vi "Leakge_Parse_Write.vi"(0 "LKG Path":path, 1 "Y2 axis on/off":bool, 2 "Y2 axis settings":T2, 3 "Vd Data":dbl[](array[numeric]), 5 "Var1 sweep settings":T3, 7 "Header in":string, 9 "Var2 step settings":T1, 11 "Vname 2":string, 12 "Execute?":bool, 13 "Vname":string, 14 "Y2 Output Cluster":cluster{"trace":dbl[], "trace":dbl[]}) -> ()   [LabVIEW 2012]
uses:
  <vilib>/Utility/file.llb/Write To Spreadsheet File (DBL).vi
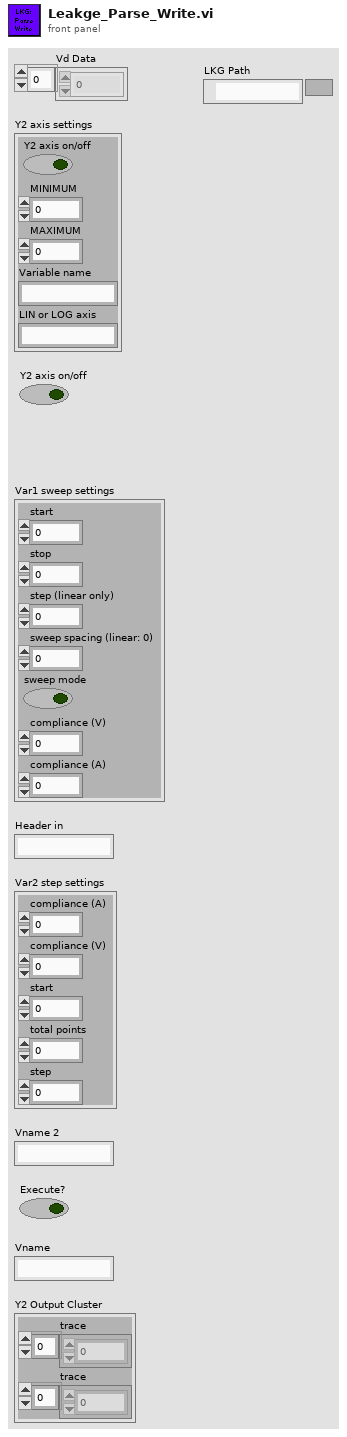
[diagram p1: front panel]
types:
  T1 = cluster{"compliance (A)":dbl, "compliance (V)":dbl, "start":dbl, "total points":u16, "step":dbl}
  T2 = cluster{"Y2 axis on/off":bool, "MINIMUM":ext, "MAXIMUM":ext, "Variable name":string, "LIN or LOG axis":string}
  T3 = cluster{"start":dbl, "stop":dbl, "step (linear only)":dbl, "sweep spacing (linear: 0)":u16, "sweep mode":bool, "compliance (V)":dbl, "compliance (A)":dbl}
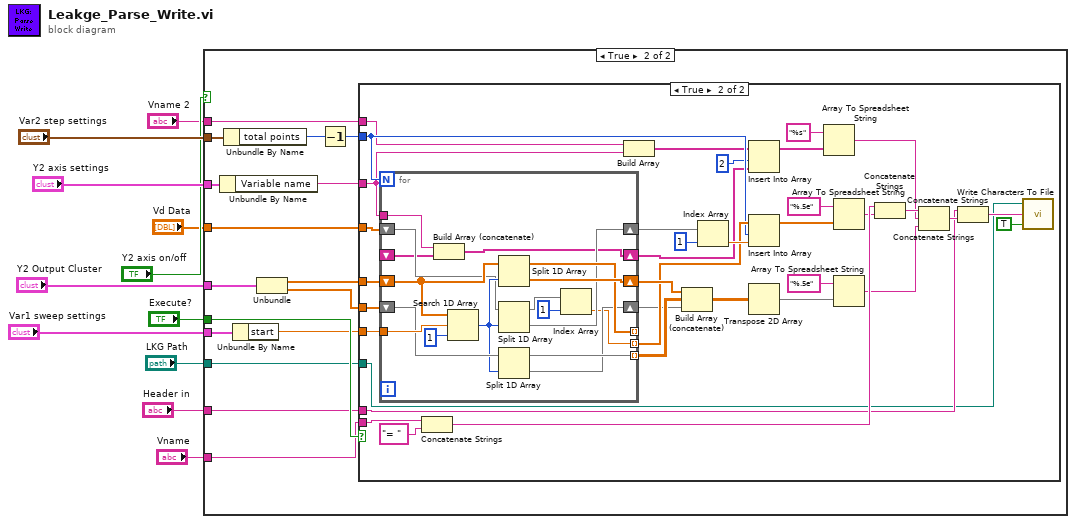
[diagram p0: block diagram]
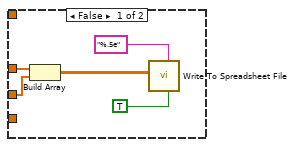
[diagram p3: hidden frame]
diagram:
  n1 = case shown="True" "Y2 axis on/off" {
    tunnel: "Execute?" -> [_ w27]
    tunnel: "Vd Data" -> [_ w26]
    tunnel: "Vname" -> [_ w25]
    tunnel: "Vname 2" -> [_ w24]
    tunnel: "Header in" -> [_ w23]
    tunnel: "LKG Path" -> [_ w22]
    tunnel: "Var2 step settings" -> [_ w21]
    tunnel: "Y2 axis settings" -> [_ w18]
    tunnel: "Var1 sweep settings" -> [_ w16]
    tunnel: "Y2 Output Cluster" -> [_ w14]
    frame False {
    }
    frame True {
      n2 = Unbundle By Name(w18) -> ("Variable name"=w17:string)
      n3 = Unbundle By Name(w21) -> ("total points"=w20:u16)
      n4 = Unbundle By Name(w16) -> ("start"=w15:dbl)
      n5 = Unbundle(w14) -> ("trace"=w13:dbl[], "trace"=w12:dbl[])
      n6 = Decrement(x=w20) -> (x-1=w19:u16)
      n7 = case shown="True" w27 {
        tunnel: w19 -> [_ w56]
        tunnel: w13 -> [w31 w68]
        tunnel: w15 -> [_ w67]
        tunnel: w12 -> [w32 w66]
        tunnel: w26 -> [_ w65]
        tunnel: w25 -> [_ w53]
        tunnel: w17 -> [_ w46]
        tunnel: w24 -> [_ w45]
        tunnel: w23 -> [_ w34]
        tunnel: w22 -> [_ w33]
        frame False {
          n8 = Build Array(w31, w32) -> (w30:dbl[][])
          n9 = call-poly <vilib>:"Write To Spreadsheet File.vi"("transpose? (no:F)"=TRUE, "format (%.3f)"="%.5e", "2D data"=w30) -> ()  [unwired: 5 in, 1 out]
        }
        frame True {
          n10 = for {
            N: w56 -> [_]
            shift-right: [w82] -> w64
            shift-left: w68 -> [w83]
            tunnel: w67 -> [w85]
            tunnel: [w81] -> _ mode=indexing
            shift-right: [w78] -> w48
            shift-left: w66 -> [w80]
            tunnel: [w79] -> w63 mode=indexing
            shift-right: [w75] -> w60
            shift-left: w65 -> [w76]
            tunnel: [w72] -> w57 mode=indexing
            shift-right: [w71] -> w47
            shift-left: _ -> [w70]
            tunnel: w46 -> [w69]
            n11 = Build Array (concatenate)(w69, w70) -> (w71:string[])
            n12 = Search 1D Array(1D array=w83, element=w85, start index (0)=1) -> (index of element=w77:i32)
            n13 = Split 1D Array(array=w83, index=w77) -> (first subarray=w81:dbl[], second subarray=w82:dbl[])
            n14 = Split 1D Array(array=w76, index=w77) -> (first subarray=w73:dbl[], second subarray=w75:dbl[])
            n15 = Split 1D Array(array=w80, index=w77) -> (first subarray=w79:dbl[], second subarray=w78:dbl[])
            n16 = Index Array(array=w73, index=1) -> (element=w72:dbl)
          }
          n17 = Concatenate Strings(w53, "= " ("string")) -> (w43:string)
          n18 = Build Array(w45, w46) -> (w50:string[])
          n19 = Build Array (concatenate)(w64, w63, w48) -> (w62:dbl[][])
          n20 = Index Array(array=w60, index=1) -> (element=w58:dbl)
          n21 = Insert Into Array(array=w50, index=2, new element=w47) -> (w49:string[])
          n22 = Insert Into Array(array=w57, index=w56, new element=w58) -> (w55:dbl[])
          n23 = Transpose 2D Array(2D array=w62) -> (transposed array=w61:dbl[][])
          n24 = Array To Spreadsheet String(array=w49, 3:"%s") -> (spreadsheet string=w39:string)  [unwired: 1 in]
          n25 = Array To Spreadsheet String(array=w55, 3:"%.5e" ("format string")) -> (spreadsheet string=w42:string)  [unwired: 1 in]
          n26 = Array To Spreadsheet String(array=w61, 3:"%.5e" ("format string")) -> (spreadsheet string=w40:string)  [unwired: 1 in]
          n27 = Concatenate Strings(w43, w42) -> (w41:string)
          n28 = Concatenate Strings(w41, w39, w40) -> (w35:string)
          n29 = Concatenate Strings(w34, w35) -> (w36:string)
          n30 = call <vilib>:"Write Characters To File.vi"("append to file? (new file:F)"=TRUE, "character string"=w36, "file path (dialog if empty)"=w33) -> ()  [unwired: 2 in, 1 out]
        }
      }
    }
  }
